vi "Log.vi"   [LabVIEW 2011, in "Konvolucio MUDS150628.lvlib"]
uses:
  <instrlib>/Konvolucio MUDS150628/Konvolucio MUDS150628.lvlib
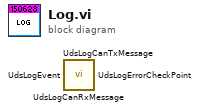
[diagram p0: block diagram]
diagram:
  n1 = call <instrlib>:"UdsLogCanRxMessage.vi"() -> ()  [unwired: 14 in, 2 out]
  n2 = call <instrlib>:"UdsLogCanTxMessage.vi"() -> ()  [unwired: 14 in, 2 out]
  n3 = call <instrlib>:"UdsLogEvent.vi"() -> ()  [unwired: 14 in, 2 out]
  n4 = call <instrlib>:"UdsLogErrorCheckPoint.vi"() -> ()  [unwired: 14 in, 2 out]
